vi "_RT_CtrlLoop_Laser_ReadStatus.vi"(6 "ExpVar in":refnum<class "ExpVar.lvclass">, 8 "error in (no error)":errorcluster, 11 "Laser349 in":refnum<class "Laser349.lvclass">) -> (0 "error out":errorcluster, 3 "Laser349 out":refnum<class "Laser349.lvclass">)   [LabVIEW 2018]
uses:
  Class/Laser349.lvclass
  PublicSubVI/NewExpVar/ExpVar.lvclass
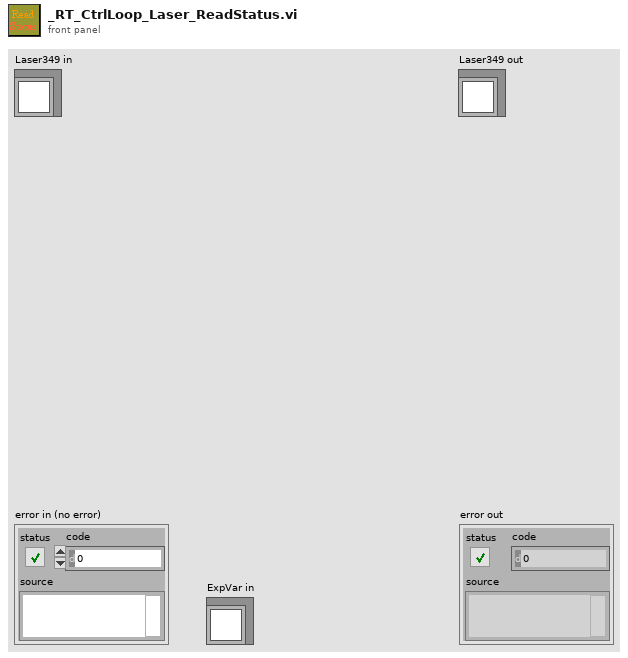
[diagram p1: front panel]
types:
  T1 = enum16{"via string label", "Laser", "Pressure", "TMP", "Script", "Signal Remarks", "ExtAO", "ExtDO", "ExtDI", "D999"}
  T2 = typedef "_ctl_LaserStatus.ctl" = cluster{"DiodeTemp":string, "SHGTemp":string, "THGTemp":string, "HeadTemp":string, "DiodeHour":string, "PulseCount":string, "PulseEnergy":string, "Actual Freq":string, "Actual Current%":string, "Actual Current Max":string, "SystemStatus":string, "Error":string}
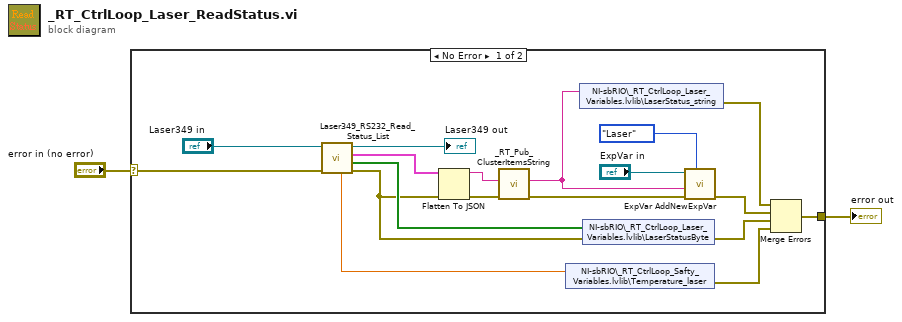
[diagram p0: block diagram]
diagram:
  n1 = case shown="No Error" "error in (no error)" {
    selector: "error in (no error)" -> [w3 w21]
    tunnel: [w10 w21] -> w2
    frame No Error {
      n2 = call-dynamic "Laser349_RS232_Read_Status_List.vi"("error in (no error)"=w3, "Laser349 in"="Laser349 in") -> ("error out"=w11:errorcluster, "Boolean array"=w19:bool[], "Laser_349_status"=w14:T2, "Laser349 out"=→"Laser349 out":refnum<class "Laser349.lvclass">, "Temperature_Laser_Value"=w18:sgl)  [unwired: 5 in]
      n3 = Flatten To JSON(anything=w14, error in (no error)=w11) -> (JSON string=w12:string, 11:w20:errorcluster)  [unwired: 1 in]
      n4 = call "_RT_Pub_ClusterItemsString.vi"("error in (no error)"=w20, "JSON string"=w12) -> ("error out"=w7:errorcluster, "result string"=w5:string)  [unwired: 8 in]
      n5 = shared-variable "NI-sbRIO\\_RT_CtrlLoop_Safty_Variables.lvlib\\Temperature_laser"(w18) -> (error out=w13:errorcluster)  [unwired: 1 in]
      n6 = shared-variable "NI-sbRIO\\_RT_CtrlLoop_Laser_Variables.lvlib\\LaserStatus_string"(w5) -> (error out=w4:errorcluster)  [unwired: 1 in]
      n7 = shared-variable "NI-sbRIO\\_RT_CtrlLoop_Laser_Variables.lvlib\\LaserStatusByte"(w19, error in=w11) -> (error out=w17:errorcluster)
      n8 = call-dynamic "ExpVar AddNewExpVar.vi"("VarType"=T1."Laser", "error in (no error)"=w7, "Var"=w5, "ExpVar in"="ExpVar in") -> ("error out"=w6:errorcluster)  [unwired: 6 in, 1 out]
      n9 = Merge Errors(w4, w6, w17, w13) -> (w10:errorcluster)
    }
    frame Error {
    }
  }
  "error out" <- w2
